vi "FetchData.vi"(8 "error in (no error)":errorcluster, 10 "Num_Records (0 for all)":u32, 11 "OXY_SCPI Reseource In":refnum<visa-resource-name>) -> (0 "error out":errorcluster, 1 "communication_data":T1, 2 "Raw Data Stream":string, 3 "OXY_SCPI Reseource Out":refnum<visa-resource-name>)   [LabVIEW 2018, in "OXYGEN.lvlib"]
doc: "Fetches MAX_RECORDS records or less from the internal ELOG buffer. If no parameter is given, all available records are returned. FETCh is only possible after STARt."
uses:
  OXYGEN.lvlib
  TypeDefs/Cluster_RawCommData.ctl
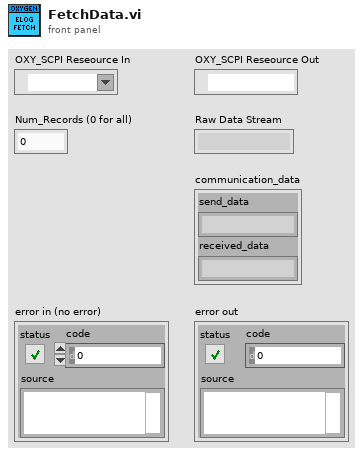
[diagram p1: front panel]
types:
  T1 = typedef "OXYGEN.lvlib/Cluster_RawCommData.ctl" = cluster{"send_data":string, "received_data":string}
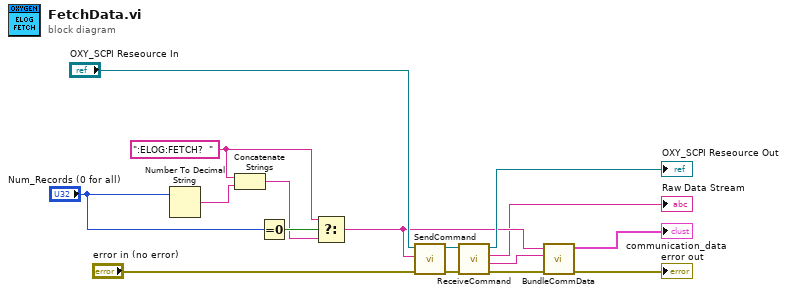
[diagram p0: block diagram]
diagram:
  w6 = ":ELOG:FETCH?  " ("string")
  n1 = Number To Decimal String(number="Num_Records (0 for all)") -> (decimal integer string=w8:string)  [unwired: 1 in]
  n2 = Concatenate Strings(w6, w8) -> (w5:string)
  n3 = Equal To 0?(x="Num_Records (0 for all)") -> (x = 0?=w7:bool)
  n4 = Select(t=w6, s=w7, f=w5) -> (s? t:f=w4:string)
  n5 = call "SendCommand.vi"("error in (no error)"="error in (no error)", "String to Send"=w4, "OXY_SCPI Reseource In"="OXY_SCPI Reseource In") -> ("error out"=w10:errorcluster, "OXY_SCPI Reseource Out"=w11:refnum<visa-resource-name>)  [unwired: 7 in]
  n6 = call "ReceiveCommand.vi"("error in (no error)"=w10, "OXY_SCPI Reseource In"=w11) -> ("error out"=w3:errorcluster, "received Data with Header"=w13:string, "received Data"=→"Raw Data Stream":string, "OXY_SCPI Reseource Out"=→"OXY_SCPI Reseource Out":refnum<visa-resource-name>)  [unwired: 6 in]
  n7 = call "BundleCommData.vi"("error in (no error)"=w3, "received_data"=w13, "send_data"=w4) -> ("error out"=→"error out":errorcluster, "communication_data"=→"communication_data":T1)  [unwired: 7 in]
